vi "LUCS001RT_GPS_Processor_ReadNumberOfBytes.vi"(6 "stop":bool, 7 "timeout in ms (-1)":i32=1000, 8 "error in":errorcluster, 10 "BytesToRad":i32, 11 "GPS Queue":refnum<queue>) -> (0 "error out":errorcluster, 1 "SerialData":string, 3 "GPS Queue DUP":refnum<queue>)   [LabVIEW 2020]
panel:
  out "TimedOut":bool
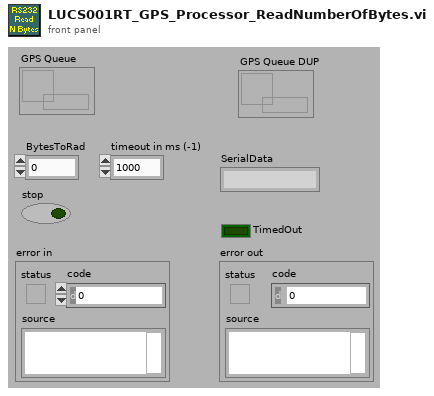
[diagram p1: front panel]
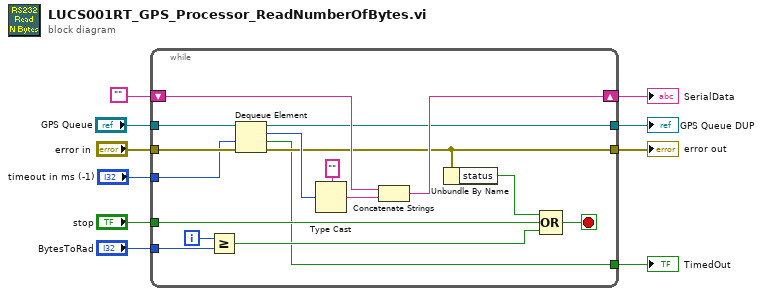
[diagram p0: block diagram]
diagram:
  n1 = while {
    tunnel: "error in" -> [w17]
    shift-right: [w25] -> w9
    shift-left: "" -> [w26]
    tunnel: [w14] -> w8
    tunnel: "stop" -> [w22]
    tunnel: "BytesToRad" -> [w20]
    tunnel: [w13] -> w4
    tunnel: "GPS Queue" -> [w16]
    tunnel: [w12] -> w2
    tunnel: "timeout in ms (-1)" -> [w11]
    i -> [w21]
    stop <- w27 stop-if-true
    n2 = Greater Or Equal?(x=w21, y=w20) -> (x >= y?=w19:bool)
    n3 = Dequeue Element(queue=w16, timeout in ms (-1)=w11, error in (no error)=w17) -> (queue out=w12:refnum<queue>, element=w15:u8, timed out?=w13:bool, error out=w14:errorcluster)
    n4 = Type Cast(type="", x=w15) -> (*(type *) &x=w23:string)
    n5 = Concatenate Strings(w26, w23) -> (w25:string)
    n6 = Unbundle By Name(w14) -> ("status"=w24:bool)
    n7 = Compound Arithmetic op=OR(w24, w22, w19) -> (w27:bool)
  }
  "SerialData" <- w9
  "error out" <- w8
  "TimedOut" <- w4
  "GPS Queue DUP" <- w2
